vi "Periodic Tasks.vi"(8 "error in":errorcluster) -> ()   [LabVIEW 2014]
doc: "This VI runs in parallel to other tasks. It can contain as many user-defined periodic loops as you need. These can carry out PID or other sorts of timed response."
uses:
  <vilib>/Rock Robotics/SystemInterfaces/Utilities/FPGA_UtilitiesLED Source.ctl
  <vilib>/Rock Robotics/SystemInterfaces/Utilities/FPGA_UtilitiesLED State.ctl
  Robot Global Data.vi
  <vilib>/Rock Robotics/WPI/Solenoid/WPI_SolenoidSetEnum.vi
  <vilib>/Rock Robotics/WPI/Solenoid/WPI_SolenoidValue.ctl
  <vilib>/Rock Robotics/WPI/Solenoid/WPI_SolenoidGetEnum.vi
panel:
  out ".not. x?":bool
  out "AUTONOMOUS MODE":i32
  in  "Goto Setting 4":bool
  in  "Goto Setting 3":bool
  out "Hot Target":bool
  out "Numeric":i32
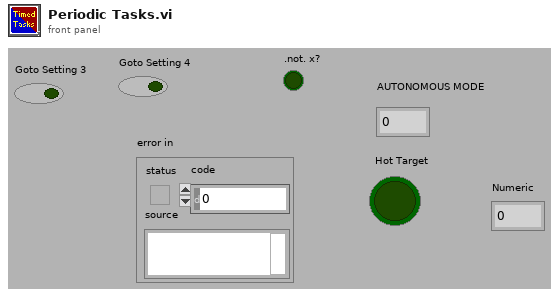
[diagram p1: front panel]
types:
  T1 = cluster{"Setting 1":dbl, "Setting 2":dbl, "Setting 3":dbl, "Setting 4":dbl, "Min":dbl, "Max":dbl}
  T2 = cluster{"Button 1":bool, "Button 2":bool, "Button 3":bool, "Button 4":bool, "Invert?":bool}
  T3 = typedef "WPI_RobotDriveDevRef.ctl" = cluster{"DevStatus":errorcluster, "Motors[]":T4[], "Square Inputs":bool, "Max Output":dbl}
  T4 = typedef "WPI_MotorControlDeviceRef.ctl" = cluster{"DeviceStatus":errorcluster, "Type":T5, "PWM":cluster{"Controller":T6, "PWM Channel":T7, "DeadBand":T8}, "CAN":cluster{"Device Number":u8, "Control Mode":T9, "Semaphore":T10, "Max Vout":dbl, "TalonSRX Control Mode":T11}, "Invert":bool, "TransformRef":T12, "InvTransformRef":T12}
  T5 = typedef "WPI_MotorControlType.ctl" = enum16{"PWM", "CAN", "CANTalonSRX"}
  T6 = typedef "FPGA_TypedefDigitalModule.ctl" = enum16{"Controller 1"}
  T7 = typedef "FPGA_DIOPWMChannel.ctl" = enum8{"PWM 0", "PWM 1", "PWM 2", "PWM 3", "PWM 4", "PWM 5", "PWM 6", "PWM 7", "PWM 8", "PWM 9", "PWM MXP 0", "PWM MXP 1", "PWM MXP 2", "PWM MXP 3", "PWM MXP 4", "PWM MXP 5", "PWM MXP 6", "PWM MXP 7", "PWM MXP 8", "PWM MXP 9", "Invalid"}
  T8 = typedef "WPI_PWMDeadband.ctl" = cluster{"Name":string, "maxPositivePwm":i32, "minPositivePwm":i32, "centerPwm":i32, "maxNegativePwm":i32, "minNegativePwm":i32, "angularRange":u16}
  T9 = typedef "WPI_CANJaguar_ControlMode.ctl" = enum8{"Percent VBus", "Current", "Speed", "Position", "Voltage"}
  T10 = typedef "Semaphore RefNum" = refnum<k1>
  T11 = typedef "WPI_CANTalonSRX_APIControlMode.ctl" = enum8{"Percent VBus", "Speed", "Position", "Slave", "Unchanged / Invalid"}
  T12 = typedef "WPI_PWMTransform_ConPane.ctl" = refnum<vi>
  T13 = typedef "WPI_JoystickDevRef.ctl" = cluster{"Device":T14}
  T14 = typedef "WPI_JoystickDeviceEnum.ctl" = enum16{"USB 0", "USB 1", "USB 2", "USB 3", "USB 4", "USB 5"}
  T15 = cluster{"JoystickDevRef":T13, "RobotDriveDevRef":T3}
  T16 = typedef "WPI_SolenoidDevRef.ctl" = cluster{"DevStatus":errorcluster, "Pneumatics Control Module":u8, "Forward Solenoid Channel":T17, "Reverse Solenoid Channel":T17}
  T17 = typedef "WPI_SolenoidChannel.ctl" = enum8{"Solenoid 0", "Solenoid 1", "Solenoid 2", "Solenoid 3", "Solenoid 4", "Solenoid 5", "Solenoid 6", "Solenoid 7", "Invalid"}
  T18 = typedef "WPI_AnalogChannelDevRef.ctl" = cluster{"DevStatus":errorcluster, "Controller":T19, "Analog Channel":T20}
  T19 = typedef "FPGA_TypedefAnalogModule.ctl" = enum16{"Controller 1"}
  T20 = typedef "FPGA_AIChannel.ctl" = enum8{"AI 0", "AI 1", "AI 2", "AI 3", "AI MXP 0", "AI MXP 1", "AI MXP 2", "AI MXP 3", "Invalid"}
  T21 = typedef "WPI_SolenoidValue.ctl" = enum16{"Off", "On", "Forward", "Reverse"}
  T22 = cluster{"Button 1":bool, "Button 2":bool, "Button 3":bool, "Button 4":bool, "Button 5":bool, "Button 6":bool, "Button 7":bool, "Button 8":bool, "Button 9":bool, "Button 10":bool, "Button 11":bool, "Button 12":bool}
  T23 = cluster{"axis 1 (x)":dbl, "axis 2 (y)":dbl, "axis 3 (throttle)":dbl, "axis 4":dbl, "axis 5":dbl, "axis 6":dbl}
  T24 = typedef "FPGA_UtilitiesLED State.ctl" = enum16{"Off", "On", "Toggle"}
  T25 = typedef "FPGA_UtilitiesLED Source.ctl" = enum16{"User LED", "FPGA LED"}
  T26 = typedef "WPI_CompressorDevRef.ctl" = cluster{"DevStatus":errorcluster, "Pneumatics Control Module":u8}
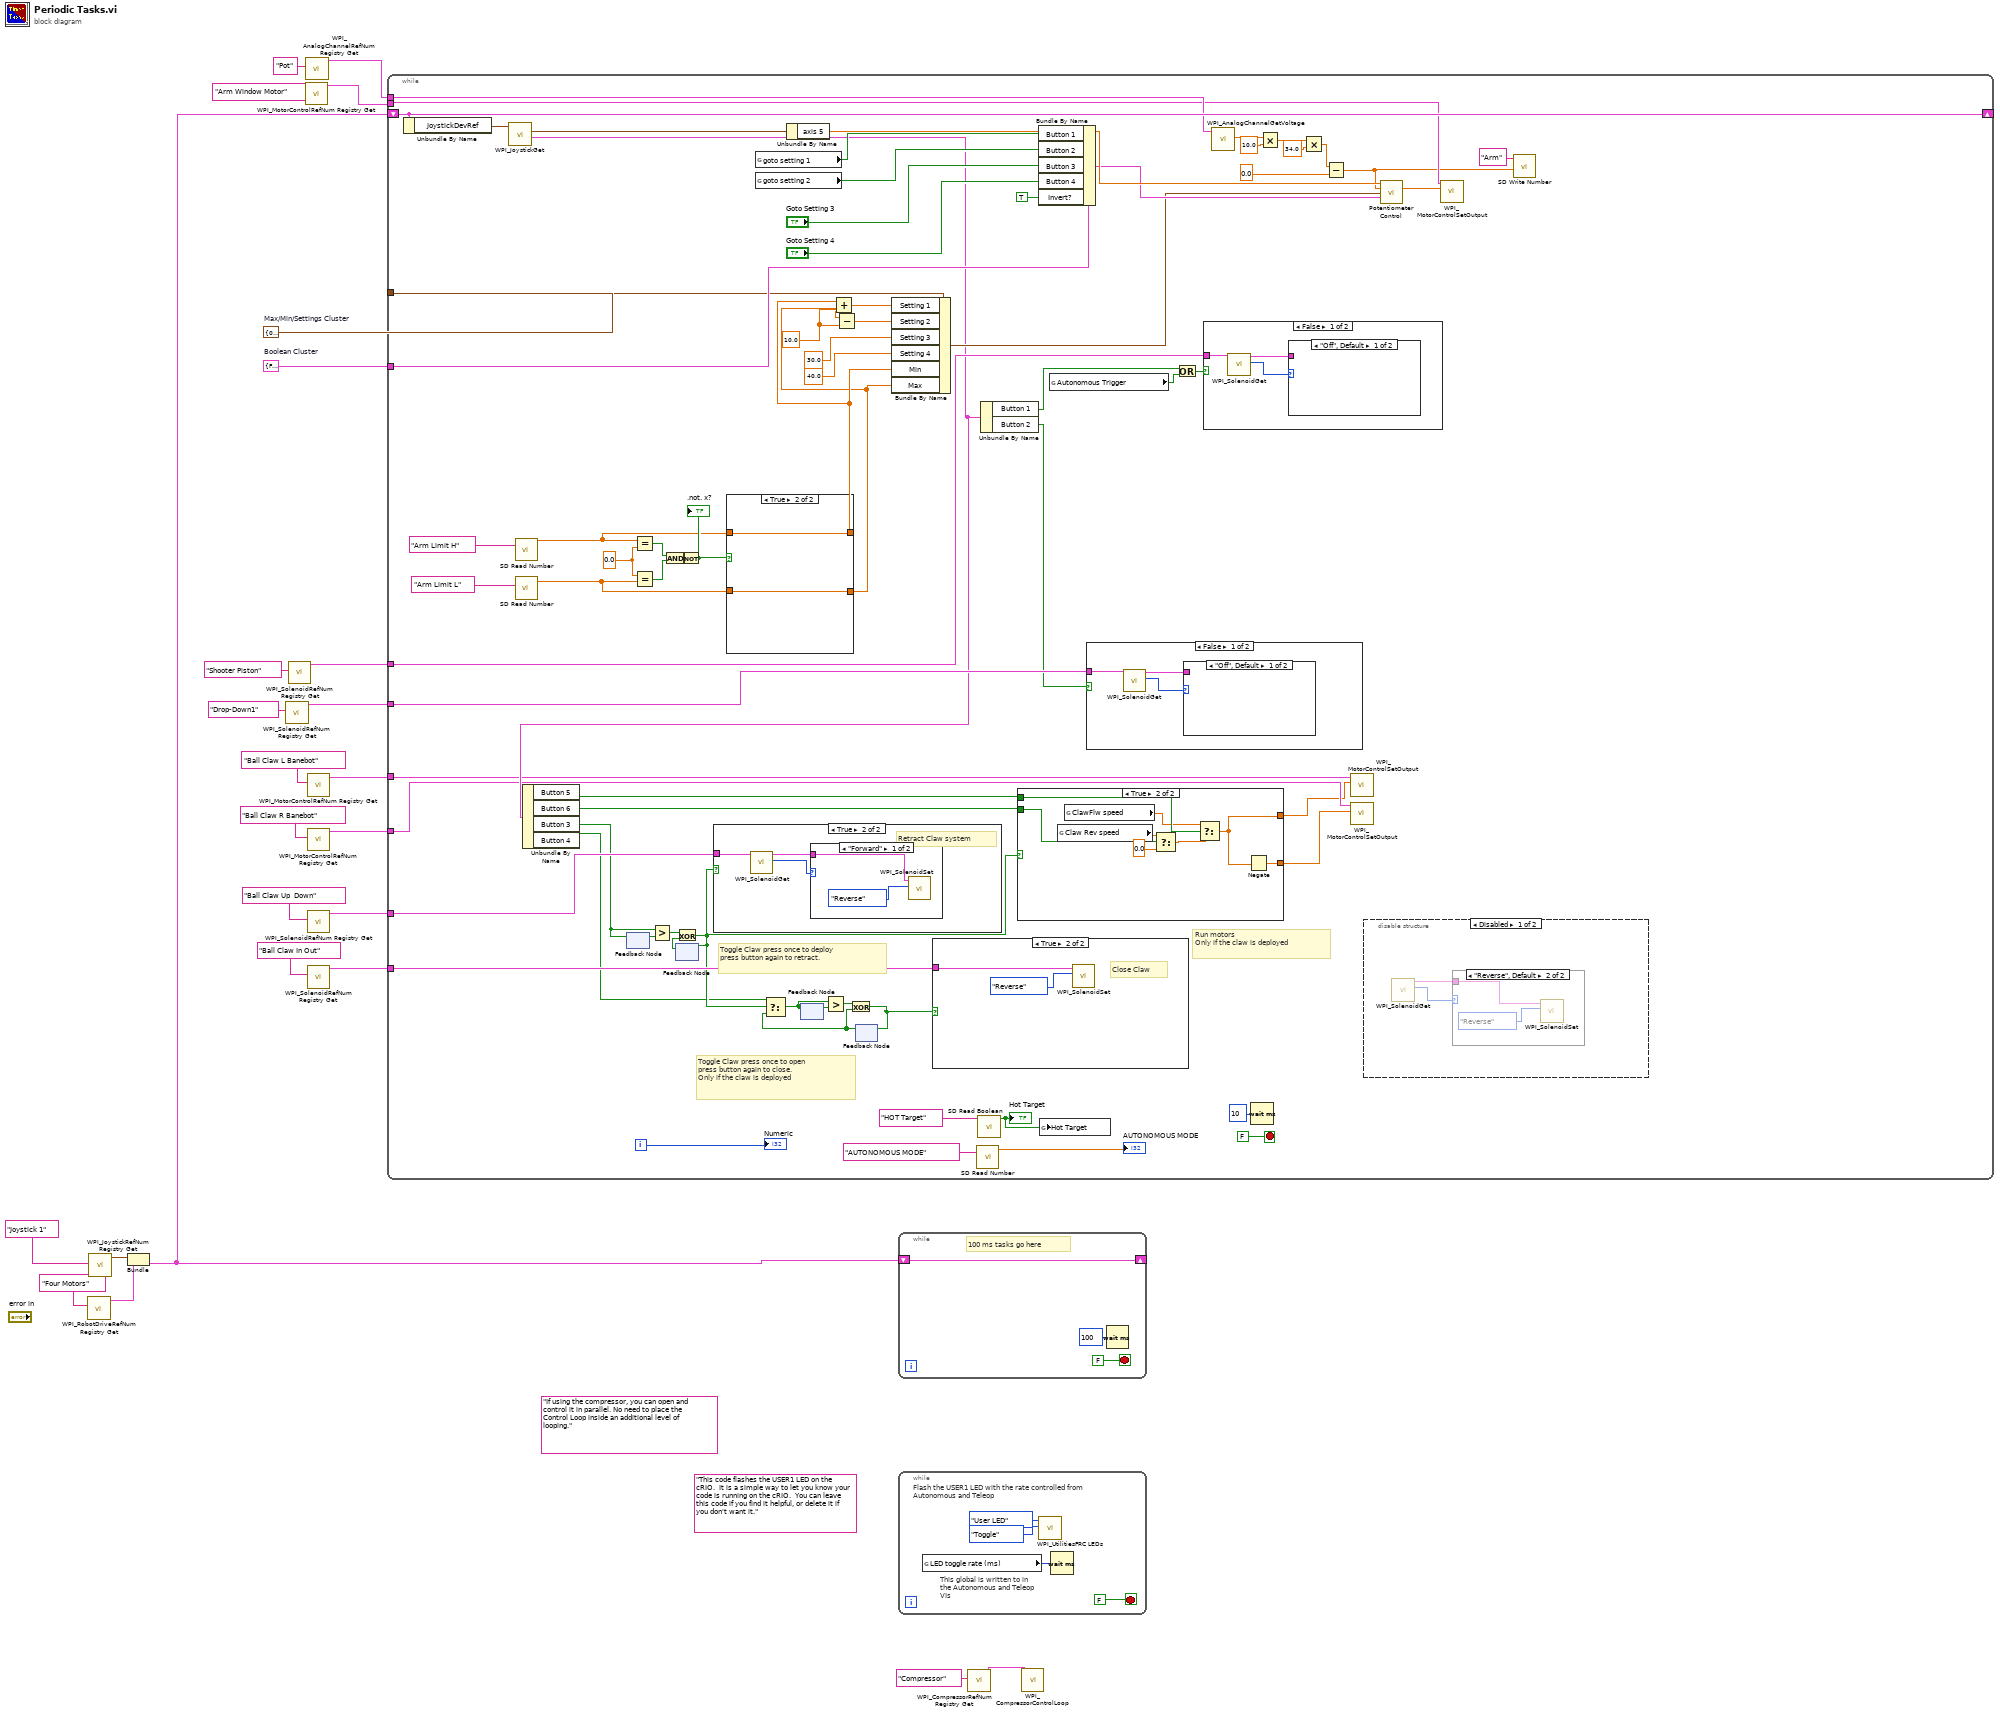
[diagram p0: block diagram]
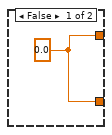
[diagram p4: hidden frame]
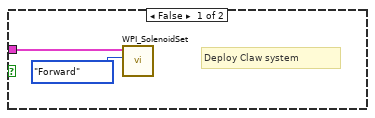
[diagram p5: hidden frame]
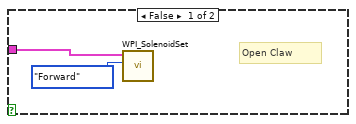
[diagram p7: hidden frame]
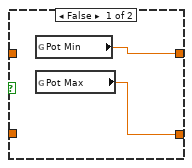
[diagram p8: hidden frame]
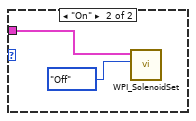
[diagram p9: hidden frame]
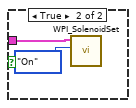
[diagram p10: hidden frame]
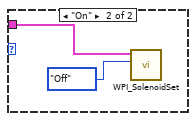
[diagram p11: hidden frame]
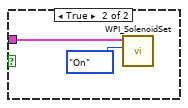
[diagram p12: hidden frame]
diagram:
  w17 = T1 {"Setting 1"=0.0, "Setting 2"=0.0, "Setting 3"=0.0, "Setting 4"=0.0, "Min"=0.0, "Max"=0.0}  # Max/Min/Settings Cluster
  w18 = T2 {"Button 1"=FALSE, "Button 2"=FALSE, "Button 3"=FALSE, "Button 4"=FALSE, "Invert?"=FALSE}  # Boolean Cluster
  (unwired) "If using the compressor, you can open and control it in parallel. No need to place the Control Loop inside an additional level of looping."
  (unwired) "This code flashes the USER1 LED on the cRIO.  It is a simple way to let you know your code is running on the cRIO.  You can leave this code if you find it helpful, or delete it if you don't want it."
  n1 = call <vilib>:"WPI_RobotDriveRefNum Registry Get.vi"("refnum name"="Four Motors") -> ("RobotDriveDevRef"=w22:T3)  [unwired: 1 in, 9 out]
  n2 = call <vilib>:"WPI_JoystickRefNum Registry Get.vi"("refnum name"="Joystick 1") -> ("JoystickDevRef"=w23:T13)  [unwired: 1 in, 9 out]
  n3 = Bundle("JoystickDevRef"=w23, "RobotDriveDevRef"=w22) -> (w21:T15)  [unwired: 1 out]
  n4 = call <vilib>:"WPI_SolenoidRefNum Registry Get.vi"("refnum name"="Drop-Down1") -> ("SolenoidDevRef"=w15:T16)  [unwired: 9 in, 1 out]
  n5 = call <vilib>:"WPI_SolenoidRefNum Registry Get.vi"("refnum name"="Shooter Piston") -> ("SolenoidDevRef"=w11:T16)  [unwired: 9 in, 1 out]
  n6 = call <vilib>:"WPI_MotorControlRefNum Registry Get.vi"("refnum name"="Arm Window Motor") -> ("MotorControlDevRef"=w5:T4)  [unwired: 9 in, 1 out]
  n7 = call <vilib>:"WPI_AnalogChannelRefNum Registry Get.vi"("refnum name"="Pot") -> ("AIDeviceRef"=w10:T18)  [unwired: 9 in, 1 out]
  n8 = call <vilib>:"WPI_MotorControlRefNum Registry Get.vi"("refnum name"="Ball Claw L Banebot") -> ("MotorControlDevRef"=w4:T4)  [unwired: 9 in, 1 out]
  n9 = call <vilib>:"WPI_MotorControlRefNum Registry Get.vi"("refnum name"="Ball Claw R Banebot") -> ("MotorControlDevRef"=w3:T4)  [unwired: 9 in, 1 out]
  n10 = call <vilib>:"WPI_SolenoidRefNum Registry Get.vi"("refnum name"="Ball Claw Up  Down") -> ("SolenoidDevRef"=w2:T16)  [unwired: 9 in, 1 out]
  n11 = call <vilib>:"WPI_SolenoidRefNum Registry Get.vi"("refnum name"="Ball Claw In Out") -> ("SolenoidDevRef"=w1:T16)  [unwired: 9 in, 1 out]
  n12 = while {
    shift-right: [w93] -> _
    shift-left: w21 -> [w93]
    tunnel: w18 -> [w90]
    tunnel: w17 -> [w87]
    tunnel: w15 -> [w83]
    tunnel: w11 -> [w82]
    tunnel: w10 -> [w75]
    tunnel: w5 -> [w74]
    tunnel: w4 -> [w39]
    tunnel: w3 -> [w38]
    tunnel: w2 -> [w45]
    tunnel: w1 -> [w40]
    i -> [w96]
    stop <- FALSE stop-if-true
    w57 = 0.0
    w61 = 10.0
    # "Run motors\nOnly if the claw is deployed"
    # "Toggle Claw press once to deploy\npress button again to retract."
    # "Toggle Claw press once to open\npress button again to close.\nOnly if the claw is deployed"
    n13 = Unbundle By Name(w93) -> ("JoystickDevRef"=w92:T13)
    n14 = call <vilib>:"WPI_JoystickGet.vi"("JoystickDevRef"=w92) -> ("Buttons"=w44:T22, "Axes"=w91:T23)  [unwired: 4 in, 1 out]
    n15 = call <vilib>:"SD Read Number.vi"("Name"="Arm Limit H") -> ("Numeric"=w52:dbl)  [unwired: 8 in, 2 out]
    n16 = call <vilib>:"SD Read Number.vi"("Name"="Arm Limit L") -> ("Numeric"=w51:dbl)  [unwired: 8 in, 2 out]
    n17 = Unbundle By Name(w44) -> ("Button 5"=w34:bool, "Button 6"=w33:bool, "Button 3"=w37:bool, "Button 4"=w29:bool)
    n18 = feedback #1() -> (w43:bool)  [unwired: 1 in]
    n19 = feedback-in #1(w37) -> ()
    n20 = Equal?(x=w52, y=w57) -> (x = y?=w56:bool)
    n21 = Equal?(x=w57, y=w51) -> (x = y?=w55:bool)
    n22 = Greater?(x=w37, y=w43) -> (0:w42:bool)
    n23 = And(x=w56, y=w55) -> (x .and. y?=w54:bool)
    n24 = feedback #2() -> (w41:bool)  [unwired: 1 in]
    n25 = Exclusive Or(1:w41, 2:w42) -> (0:w30:bool)
    n26 = feedback-in #2(w30) -> ()
    n27 = Not(x=w54) -> (.not. x?=w53:bool)
    ".not. x?" <- w53
    n28 = case shown="True" w30 {
      tunnel: w45 -> [w113 w116]
      frame False {
        # "Deploy Claw system"
        n29 = call-poly <vilib>:"WPI_SolenoidSet.vi"("Value"=WPI_SolenoidValue."Forward", "SolenoidDevRef"=w113) -> ()  [unwired: 8 in, 2 out]
      }
      frame True {
        # "Retract Claw system"
        n30 = call-poly <vilib>:"WPI_SolenoidGet.vi"("SolenoidDevRef"=w116) -> ("Value"=w114:T21, "SolenoidDevRef"=w115:T16)  [unwired: 8 in, 1 out]
        n31 = case shown="\"Forward\"" w114 {
          tunnel: w115 -> [w117 _]
          frame "Forward" {
            n32 = call-poly <vilib>:"WPI_SolenoidSet.vi"("Value"=WPI_SolenoidValue."Reverse", "SolenoidDevRef"=w117) -> ()  [unwired: 8 in, 2 out]
          }
          frame "Reverse", Default {
          }
        }
      }
    }
    n33 = case shown="True" w53 {
      tunnel: [w124 w126] -> w48
      tunnel: [w123 w125] -> w47
      tunnel: w52 -> [_ w126]
      tunnel: w51 -> [_ w125]
      frame False {
        n34 = global read "Robot Global Data.vi" "Pot Min"() -> (w124:dbl)
        n35 = global read "Robot Global Data.vi" "Pot Max"() -> (w123:dbl)
      }
      frame True {
      }
    }
    n36 = global read "Robot Global Data.vi" "goto setting 1"() -> (w50:bool)
    n37 = global read "Robot Global Data.vi" "goto setting 2"() -> (w49:bool)
    n38 = Unbundle By Name(w91) -> ("axis 5"=w89:dbl)
    n39 = feedback #3() -> (w32:bool)  [unwired: 1 in]
    n40 = Add(x=w48, y=w61) -> (x+y=w62:dbl)
    n41 = Subtract(x=w47, y=w61) -> (x-y=w60:dbl)
    n42 = feedback #4() -> (w26:bool)  [unwired: 1 in]
    n43 = Select(t=w29, s=w30, f=w26) -> (s? t:f=w28:bool)
    n44 = feedback-in #3(w28) -> ()
    n45 = Greater?(x=w28, y=w32) -> (0:w31:bool)
    n46 = Exclusive Or(1:w26, 2:w31) -> (0:w27:bool)
    n47 = feedback-in #4(w27) -> ()
    n48 = Bundle By Name(cluster=w87, "Setting 1"=w62, "Setting 2"=w60, "Setting 3"=30.0, "Setting 4"=40.0, "Min"=w48, "Max"=w47) -> (w86:T1)
    n49 = case shown="True" w27 {
      tunnel: w40 -> [w120 w121]
      frame False {
        # "Open Claw"
        n50 = call-poly <vilib>:"WPI_SolenoidSet.vi"("Value"=WPI_SolenoidValue."Forward", "SolenoidDevRef"=w120) -> ()  [unwired: 8 in, 2 out]
      }
      frame True {
        # "Close Claw"
        n51 = call-poly <vilib>:"WPI_SolenoidSet.vi"("Value"=WPI_SolenoidValue."Reverse", "SolenoidDevRef"=w121) -> ()  [unwired: 8 in, 2 out]
      }
    }
    n52 = call <vilib>:"SD Read Number.vi"("Name"="AUTONOMOUS MODE") -> ("Numeric"=→"AUTONOMOUS MODE":dbl)  [unwired: 8 in, 2 out]
    n53 = call <vilib>:"SD Read Boolean.vi"("Name"="HOT Target") -> ("Boolean"=w94:bool)  [unwired: 8 in, 2 out]
    "Hot Target" <- w94
    n54 = Unbundle By Name(w44) -> ("Button 1"=w66:bool, "Button 2"=w46:bool)
    n55 = case shown="True" w30 {
      tunnel: [w103 w105] -> w36
      tunnel: [w103 w104] -> w35
      tunnel: w34 -> [_ w109]
      tunnel: w33 -> [_ w108]
      frame False {
        w103 = 0.0
      }
      frame True {
        n56 = global read "Robot Global Data.vi" "Claw Rev speed"() -> (w106:dbl)
        n57 = global read "Robot Global Data.vi" "ClawFlw speed"() -> (w107:dbl)
        n58 = Select(t=w106, s=w108, f=0.0) -> (s? t:f=w111:dbl)
        n59 = Select(t=w107, s=w109, f=w111) -> (s? t:f=w104:dbl)
        n60 = Negate(x=w104) -> (-x=w105:dbl)
      }
    }
    n61 = Bundle By Name(cluster=w90, "Button 1"=w50, "Button 2"=w49, "Button 3"="Goto Setting 3", "Button 4"="Goto Setting 4", "Invert?"=TRUE) -> (w88:T2)
    n62 = global write "Robot Global Data.vi" "Hot Target"(w94) -> ()
    n63 = global read "Robot Global Data.vi" "Autonomous Trigger"() -> (w67:bool)
    n64 = case shown="False" w46 {
      tunnel: w83 -> [w136 w140]
      frame False {
        n65 = call-poly <vilib>:"WPI_SolenoidGet.vi"("SolenoidDevRef"=w136) -> ("Value"=w135:T21, "SolenoidDevRef"=w134:T16)  [unwired: 8 in, 1 out]
        n66 = case shown="\"Off\", Default" w135 {
          tunnel: w134 -> [_ w138]
          frame "Off", Default {
          }
          frame "On" {
            n67 = call-poly <vilib>:"WPI_SolenoidSet.vi"("Value"=WPI_SolenoidValue."Off", "SolenoidDevRef"=w138) -> ()  [unwired: 8 in, 2 out]
          }
        }
      }
      frame True {
        n68 = call-poly <vilib>:"WPI_SolenoidSet.vi"("Value"=WPI_SolenoidValue."On", "SolenoidDevRef"=w140) -> ()  [unwired: 8 in, 2 out]
      }
    }
    n69 = Or(x=w66, y=w67) -> (x .or. y?=w65:bool)
    n70 = case shown="False" w65 {
      tunnel: w82 -> [w129 w133]
      frame False {
        n71 = call-poly <vilib>:"WPI_SolenoidGet.vi"("SolenoidDevRef"=w129) -> ("Value"=w128:T21, "SolenoidDevRef"=w127:T16)  [unwired: 8 in, 1 out]
        n72 = case shown="\"Off\", Default" w128 {
          tunnel: w127 -> [_ w131]
          frame "Off", Default {
          }
          frame "On" {
            n73 = call-poly <vilib>:"WPI_SolenoidSet.vi"("Value"=WPI_SolenoidValue."Off", "SolenoidDevRef"=w131) -> ()  [unwired: 8 in, 2 out]
          }
        }
      }
      frame True {
        n74 = call-poly <vilib>:"WPI_SolenoidSet.vi"("Value"=WPI_SolenoidValue."On", "SolenoidDevRef"=w133) -> ()  [unwired: 8 in, 2 out]
      }
    }
    n75 = call <vilib>:"WPI_AnalogChannelGetVoltage.vi"("AIDeviceRef"=w75) -> ("Voltage"=w79:dbl)  [unwired: 8 in, 2 out]
    n76 = Wait (ms)(milliseconds to wait=u32 10) -> ()  [unwired: 1 out]
    n77 = Multiply(x=w79, y=10.0) -> (x*y=w78:dbl)
    n78 = Multiply(x=w78, y=34.0) -> (x*y=w77:dbl)
    n79 = Subtract(x=w77, y=0.0) -> (x-y=w69:dbl)
    n80 = call <vilib>:"WPI_MotorControlSetOutput.vi"("Output"=w35, "MotorControlDevRef"=w39) -> ()  [unwired: 7 in, 3 out]
    n81 = call <vilib>:"WPI_MotorControlSetOutput.vi"("Output"=w36, "MotorControlDevRef"=w38) -> ()  [unwired: 7 in, 3 out]
    n82 = disable-structure shown="Disabled" {
      frame Disabled {
        n83 = call-poly <vilib>:"WPI_SolenoidGet.vi"() -> ("Value"=w100:T21, "SolenoidDevRef"=w99:T16)  [unwired: 9 in, 1 out]
        n84 = case shown="\"Reverse\", Default" w100 {
          tunnel: w99 -> [_ w102]
          frame "Forward" {
          }
          frame "Reverse", Default {
            n85 = call-poly <vilib>:"WPI_SolenoidSet.vi"("Value"=WPI_SolenoidValue."Reverse", "SolenoidDevRef"=w102) -> ()  [unwired: 8 in, 2 out]
          }
        }
      }
      frame Enabled {
      }
    }
    n86 = call "Potentiometer Control.vi"("Arm Window Axis"=w89, "Potentiometer Input"=w69, "Max/Min/Settings Cluster"=w86, "Boolean Cluster"=w88) -> ("Output Motor Speed"=w70:dbl)  [unwired: 11 in]
    n87 = call <vilib>:"WPI_MotorControlSetOutput.vi"("Output"=w70, "MotorControlDevRef"=w74) -> ()  [unwired: 7 in, 3 out]
    n88 = call <vilib>:"SD Write Number.vi"("Numeric"=w69, "Name"="Arm") -> ()  [unwired: 8 in, 2 out]
    "Numeric" <- w96
  }
  n89 = while {
    shift-right: [w141] -> _
    shift-left: w21 -> [w141]
    stop <- FALSE stop-if-true
    # "100 ms tasks go here"
    n90 = Wait (ms)(milliseconds to wait=u32 100) -> ()  [unwired: 1 out]
  }
  n91 = while {
    stop <- FALSE stop-if-true
    # "This global is written to in the Autonomous and Teleop VIs"
    # "Flash the USER1 LED with the rate controlled from Autonomous and Teleop"
    n92 = global read "Robot Global Data.vi" "LED toggle rate (ms)"() -> (w144:u32)
    n93 = call <vilib>:"WPI_UtilitiesFRC LEDs.vi"("State"=FPGA_UtilitiesLED_State."Toggle", "LED Type"=FPGA_UtilitiesLED_Source."User LED") -> ()  [unwired: 1 in, 9 out]
    n94 = Wait (ms)(milliseconds to wait=w144) -> ()  [unwired: 1 out]
  }
  n95 = call <vilib>:"WPI_CompressorRefNum Registry Get.vi"("refnum name"="Compressor") -> ("CompressorDevRef"=w13:T26)  [unwired: 9 in, 1 out]
  n96 = call <vilib>:"WPI_CompressorControlLoop.vi"("CompressorDevRef"=w13) -> ()  [unwired: 11 in]
